vi "labbitMQ.vi"() -> ()   [LabVIEW 2022 SP3]
uses:
  <vilib>/Distrio/LabbitMQ/Connection/connection_parameters_cluster.ctl
  <vilib>/Distrio/LabbitMQ/Channel/exchange_type_enum.ctl
  <vilib>/Distrio/LabbitMQ/Connection/Connection.lvclass
  <vilib>/Distrio/LabbitMQ/Channel/Channel.lvclass
  <vilib>/Distrio/LabbitMQ/Exchange/Exchange.lvclass
panel:
  in  "Routing key":string
  in  "Message":string="{ \n    \"type\": \"sample\",\n    \"data\": {\n        id: 984658168FER4654,\n        projectId: 2000146,\n        voucherId: #26413,\n        speciesName: Spider,\n        collectionDate: 2022-10-20,\n        sampleStation: Denmark,\n        location: Denmark, \n        lat: 10.200806,\n        lon: 56.144019,\n        determiner: MRJ,\n        sex: Male,\n        exposureTime: 2000,\n        framerate: 50,\n        lightIntensityPct: 100,\n        aperture: 8,\n        operatorName: MRJ,\n        date: 2022-20-10,\n        otherNotes: TestPackage\n    }\n}"
  in  "Exchange name":string="logs"
  in  "Exchange type":T1
  in  "Connection Parameters":T2={"host name"="localhost", "port"=5672, "user name"="guest", "password"="guest", "virtual host"="/"}
  # "Structure"
  # "{ \n    \"type\": \"sample\" | \"image\" | \"summary\" | \"delete\",\n    \"data\": {\n        \n    }\n}"
  # "sample Data"
  # "image Data"
  # "summary Data"
  # "delete Data"
  # "{\n        id: 984658168FER4654,\n        projectId: 2000146,\n        voucherId: #26413,\n        speciesName: Spider,\n        collectionDate: 2022-10-20,\n        sampleStation: Denmark,\n        location: Denmark, \n        lat: 10.200806,\n        lon: 56.144019,\n        determiner: MRJ,\n        sex: Male,\n        exposureTime: 2000,\n        framerate: 50,\n        lightIntensityPct: 100,\n        aperture: 8,\n        operatorName: MRJ,\n        date: 2022-20-10,\n        otherNotes: TestPackage\n    }"
  # "{\n        sampleId: 984658168FER4654,\n        speciesName: Spider,\n        date: 2022-20-10,\n        imageName: cam1_001,\n        cameraNumber: 1, \n        imageNumber: 1,\n        maxFeretDiameter: 367,\n        perimeter: 15678,\n        area: 5461,\n        holes: 453,\n        areaHoles: 5914,\n        roiLeft: 0,\n        roiTop: 50,\n        roiRight: 461,\n        roiBottom: 511\n    }"
  # "{\n        sampleId: 984658168FER4654,\n        maxFeretDiameterMax: int,\n        maxFeretDiameterMean: float,\n        maxFeretDiameterStdDev: float,\n        perimeterMean: float,\n        perimeterStdDev: float,\n        areaMean: float,\n        areaStdDev: float,\n        holesMean: float,\n        holesStdDev: float,\n        areaHolesMean: float,\n        areaHolesStdDev: float,\n        numberOfImages: int\n    }"
  # "{\n        sampleId: 984658168FER4654\n    }"
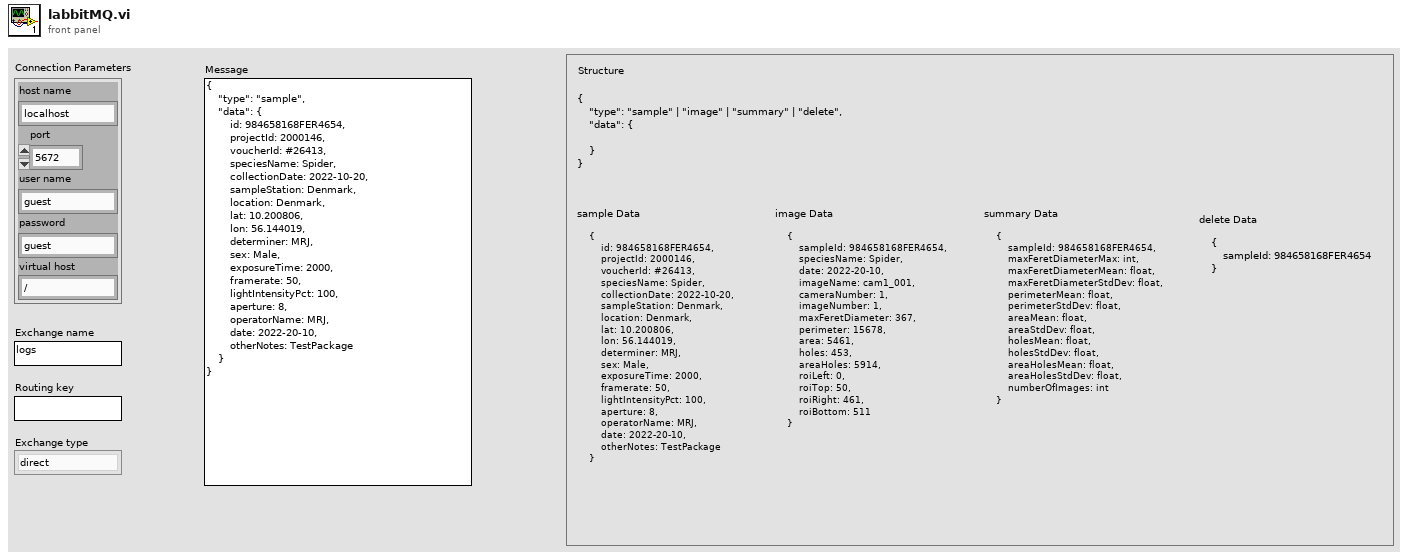
[diagram p1: front panel]
types:
  T1 = typedef "Channel.lvclass/exchange_type_enum.ctl" = enum16{"direct", "topic", "fanout", "headers"}
  T2 = typedef "Connection.lvclass/connection_parameters_cluster.ctl" = cluster{"host name":string, "port":i32, "user name":string, "password":string, "virtual host":string}
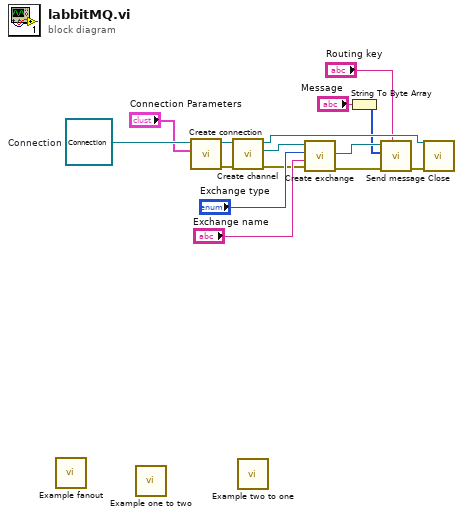
[diagram p0: block diagram]
diagram:
  w15 = refnum<class "Connection.lvclass"> refnum  # Connection
  n1 = call <vilib>:"Example fanout.vi"() -> ()  [unwired: 12 in]
  n2 = call <vilib>:"Example one to two.vi"() -> ()  [unwired: 12 in]
  n3 = call <vilib>:"Create connection.vi"("connection parameters"="Connection Parameters", "Connection in"=w15) -> ("error out"=w12:errorcluster, "Connection out"=w13:refnum<class "Connection.lvclass">)  [unwired: 8 in]
  n4 = call <vilib>:"Create channel.vi"("error in (no error)"=w12, "Connection in"=w13) -> ("error out"=w6:errorcluster, "channel"=w11:refnum<class "Channel.lvclass">, "Connection out"=w8:refnum<class "Connection.lvclass">)  [unwired: 7 in]
  n5 = call <vilib>:"Example two to one.vi"() -> ()  [unwired: 12 in]
  n6 = call <vilib>:"Create exchange.vi"("error in (no error)"=w6, "exchange name"="Exchange name", "exchange type"="Exchange type", "Channel in"=w11) -> ("error out"=w5:errorcluster, "Exchange.lvclass"=w7:refnum<class "Exchange.lvclass">)  [unwired: 5 in, 1 out]
  n7 = String To Byte Array(string="Message") -> (unsigned byte array=w3:u8[])
  n8 = call <vilib>:"Send message.vi"("routing key"="Routing key", "error in (no error)"=w5, "body"=w3, "Exchange in"=w7) -> ("error out"=w2:errorcluster)  [unwired: 6 in, 1 out]
  n9 = call <vilib>:"Close.vi"("error in (no error)"=w2, "Connection in"=w8) -> ()  [unwired: 8 in, 2 out]
